vi "HRM-P-manual_peak_detector.vi"(9 "Bot":dbl, 10 "Top":dbl, 11 "waveform in":waveform(dbl)) -> (1 "# of peaks":i32, 3 "Frequency [Hz]":dbl)   [LabVIEW 2020]
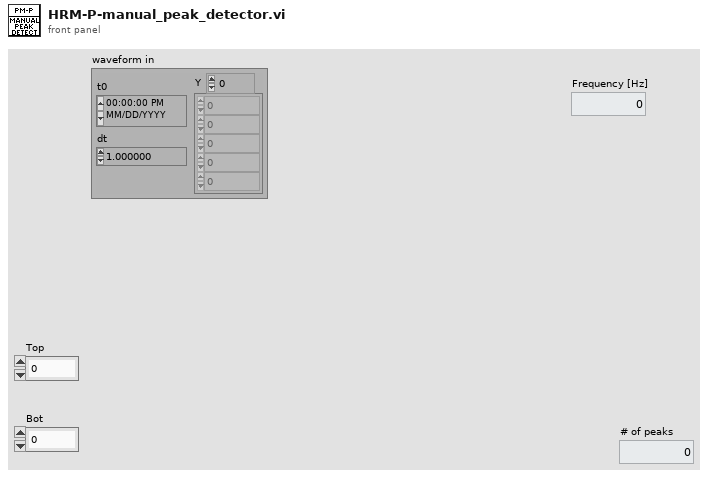
[diagram p1: front panel]
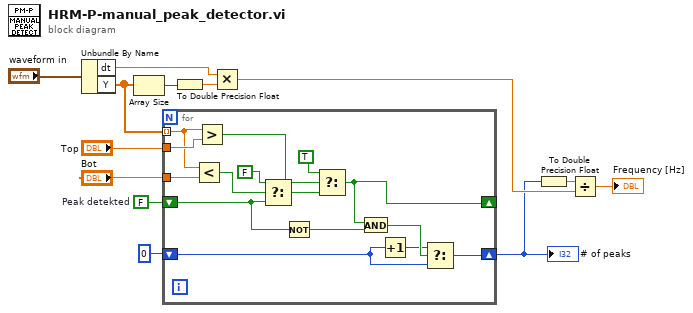
[diagram p0: block diagram]
diagram:
  w13 = FALSE  # Peak detekted
  n1 = Unbundle By Name("waveform in") -> ("dt"=w6:dbl, "Y"=w8:dbl[])
  n2 = Array Size(array=w8) -> (size(s)=w7:i32)
  n3 = for {
    tunnel: w8 -> [w27] mode=indexing
    tunnel: "Top" -> [w28]
    tunnel: "Bot" -> [w26]
    shift-right: [w18] -> _
    shift-left: w13 -> [w20]
    shift-right: [w14] -> w2
    shift-left: 0 -> [w15]
    n4 = Less?(x=w27, y=w26) -> (x < y?=w24:bool)
    n5 = Greater?(x=w27, y=w28) -> (0:w25:bool)
    n6 = Select(t=FALSE, s=w24, f=w20) -> (s? t:f=w23:bool)
    n7 = Not(x=w20) -> (.not. x?=w19:bool)
    n8 = Select(t=TRUE, s=w25, f=w23) -> (s? t:f=w18:bool)
    n9 = And(x=w18, y=w19) -> (x .and. y?=w17:bool)
    n10 = Increment(x=w15) -> (x+1=w16:i32)
    n11 = Select(t=w16, s=w17, f=w15) -> (s? t:f=w14:i32)
  }
  "# of peaks" <- w2
  n12 = To Double Precision Float(number=w7) -> (double precision float=w4:dbl)
  n13 = Multiply(x=w6, y=w4) -> (x*y=w5:dbl)
  n14 = To Double Precision Float(number=w2) -> (double precision float=w3:dbl)
  n15 = Divide(x=w3, y=w5) -> (x/y=→"Frequency [Hz]":dbl)
